vi "Main.vi"() -> ()   [LabVIEW 2013] (continued)
                                frame True {
                                # "Both FHS"
                                n2888 = Build Array(w4843, w4842) -> (w4844:refnum<vi>[])
                                }
                                }
                                n2889 = control-ref of="MCListBox FHS Setup Remove Button"() -> (w4836:refnum<vi>)
                                n2890 = control-ref of="MCListBox FHS Setup Add Button"() -> (w4837:refnum<vi>)
                                n2891 = local write "Edit WPS in Setup"(w4830) -> ()
                                n2892 = control-ref of="Tab Setup"() -> (w4839:refnum<vi>)
                                n2893 = local read "CellBG New Cells"() -> (w4832:u32)
                                n2894 = for {
                                tunnel: w4832 -> [w4849]
                                tunnel: w4835 -> [w4846] mode=indexing
                                # "MClistbox FHS Setup \nis set to FALSE for\n\"Allowing Editing Cells\"\n/\"Editable Cells"
                                # "Create WHITE\neditable cells"
                                n2895 = property on="Property Node" class="MCListbox (strict)"(reference=w4846, "Allow Editing Cells"=TRUE) -> (reference out=w4848:refnum<vi>, "NumCols"=w4847:u32)  [unwired: 1 in, 1 out]
                                n2896 = for {
                                N: w4847 -> [_]
                                tunnel: w4849 -> [w4851]
                                tunnel: w4848 -> [w4850]
                                i -> [w4853]
                                n2897 = Bundle("Multicolumn Listbox"=0, w4853) -> (w4852:cluster{"Multicolumn Listbox":i32, i32})  [unwired: 1 in]
                                n2898 = property on="Property Node" class="MCListbox (strict)"(reference=w4850, "ActiveCell"=w4852, "CellBG"=w4851) -> ()  [unwired: 1 in, 2 out]
                                }
                                }
                                n2899 = control-ref of="No."() -> (w4831:refnum<vi>)
                                n2900 = property class="Bool"(reference=w4836, "Visible"=w4830) -> ()  [unwired: 1 in, 2 out]
                                n2901 = property class="Bool"(reference=w4837, "Visible"=w4830) -> ()  [unwired: 1 in, 2 out]
                                n2902 = call "Setup Tab - Enable-Disable.vi"("No."=w4831, "[SRTRS][Config][ParameterSettings] - [userEditableProcedure]"=w4830, "Disabled"=T30."Enabled", "Tab Setup"=w4839) -> ()  [unwired: 8 in]
                              }
                            }
                            n2903 = call "DB - Convert BIT Type.vi"("BIT Type (eg Inactive)"=w4829) -> ("Boolean"=w4826:bool)  [unwired: 2 in, 2 out]
                          }
                          frame "ChartSeparation" {
                            # "Need DB - NA"
                            n2904 = call "DB - Convert BIT Type.vi"("BIT Type (eg Inactive)"=w4856) -> ("Boolean"=→"Chart Separation by Order#":bool)  [unwired: 2 in, 2 out]
                          }
                          frame "DataLogInterval" {
                            n2905 = Fract/Exp String To Number(string=w4858, default (0 dbl)=0.0) -> (number=w4860:dbl)  [unwired: 2 in, 1 out]
                            n2906 = local write "Host Sampling Interval (s)"(w4860) -> ()
                          }
                          frame "DateFormat" {
                            # "%<%H:%M:%S \n%Y-%m-%d>T"
                            n2907 = Empty String/Path?(string/path=w4862) -> (empty?=w4863:bool)
                            n2908 = case shown="False" w4863 {
                              tunnel: w4862 -> [w4868 _]
                              frame False {
                                # "We only fix time here. The date format is from DB"
                                # "Not Empty"
                                n2909 = Concatenate Strings("%<%H:%M:%S", "\n", w4868, ">T" ("string")) -> (w4867:string)
                                n2910 = property on="Chart" class="WFChart (strict)"("XScale.FormatString"=w4867) -> (error out=w4866:errorcluster)  [unwired: 2 in, 1 out]
                                n2911 = local write "Chart"(w4866) -> ()
                              }
                              frame True {
                                # "Empty"
                              }
                            }
                            "Date Format (UserDefined)" <- w4862
                          }
                          frame "EnableCmsUpdate" {
                            # "Need DB - NA"
                            n2912 = call "DB - Convert BIT Type.vi"("BIT Type (eg Inactive)"=w4873) -> ("Boolean"=w4872:bool)  [unwired: 2 in, 2 out]
                            "Enable Central Monitoring" <- w4872
                            n2913 = global write "Global SRTRS.vi" "Enable Central Monitoring"(w4872) -> ()
                          }
                          frame "EnableAmsUpdate" {
                            # "For Message UI"
                            # "No need to send to ini\nSince No DB, No AMS"
                            n2914 = call "DB - Convert BIT Type.vi"("BIT Type (eg Inactive)"=w4875) -> ("Boolean"=w4874:bool)  [unwired: 2 in, 2 out]
                            "Enable AMS Update" <- w4874
                            n2915 = global write "Global SRTRS.vi" "Enable AMS Update"(w4874) -> ()
                          }
                          frame "PermittedTempDiff" {
                            n2916 = Fract/Exp String To Number(string=w4877) -> (number=w4879:dbl)  [unwired: 3 in, 1 out]
                            n2917 = property on="Variant Allowed (Hold Temp)" class="DigNum (strict)"("Value"=w4879) -> ()  [unwired: 2 in, 2 out]
                          }
                          frame "PermittedTimeDiff" {
                            n2918 = Fract/Exp String To Number(string=w4881) -> (number=w4883:dbl)  [unwired: 3 in, 1 out]
                            n2919 = property on="Variant Allowed (Hold Time)" class="DigNum (strict)"("Value"=w4883) -> ()  [unwired: 2 in, 2 out]
                          }
                          frame "StartStopMarker" {
                            n2920 = call "DB - Convert BIT Type.vi"("BIT Type (eg Inactive)"=w4887) -> ("Boolean"=w4884:bool)  [unwired: 2 in, 2 out]
                            "Display Start Stop Marker" <- w4884
                          }
                          frame "DisplayRefChart" {
                            n2921 = call "DB - Convert BIT Type.vi"("BIT Type (eg Inactive)"=w4891) -> ("Boolean"=w4888:bool)  [unwired: 2 in, 2 out]
                            "Display Reference Chart" <- w4888
                          }
                        }
                        n2922 = case shown="\"String\"" w4798 {
                          tunnel: [w4815 w4823 w4825] -> w4804
                          tunnel: [w4814 w4822 w4824] -> w4797
                          tunnel: w4801 -> [w4813 w4821 w4825]
                          tunnel: w4803 -> [w4812 w4820 w4824]
                          tunnel: w4800 -> [w4811 w4818 _]
                          tunnel: w4799 -> [w4810 _ _]
                          tunnel: w4796 -> [_ w4817 _]
                          frame "String" {
                            n2923 = call-poly <vilib>:"Write Key.vi"("section"="Settings", "error in (no error)"=w4812, "value"=w4810, "key"=w4811, "refnum"=w4813) -> ("error out"=w4814:errorcluster, "refnum out"=w4815:T59)  [unwired: 4 in, 1 out]
                          }
                          frame "Boolean" {
                            n2924 = call-poly <vilib>:"Write Key.vi"("section"="Settings Boolean", "error in (no error)"=w4820, "value"=w4817, "key"=w4818, "refnum"=w4821) -> ("error out"=w4822:errorcluster, "refnum out"=w4823:T59)  [unwired: 4 in, 1 out]
                          }
                          frame "NA", Default {
                          }
                        }
                      }
                      n2925 = for {
                        tunnel: w4699 -> [w4760]
                        tunnel: w4698 -> [w4759]
                        tunnel: w4648 -> [w4757] mode=indexing
                        tunnel: [w4755] -> w4689
                        tunnel: [w4754] -> w4688
                        tunnel: w4709 -> [w4753]
                        tunnel: w4690 -> [w4752]
                        # "[Config].[GeneralSetting]"
                        n2926 = Format Into String(w4757) -> (resulting string=w4758:string)  [unwired: 3 in, 1 out]
                        n2927 = Search 1D Array(1D array=w4759, element=w4758) -> (index of element=w4761:i32)  [unwired: 1 in]
                        n2928 = Index Array(array=w4760, index=w4761) -> (element=w4756:string)
                        n2929 = case shown="\"TimeSyncSchedule\"" w4757 {
                          tunnel: w4756 -> [_ w4773 w4779 w4787 w4791]
                          tunnel: [_ "Log Off Timer" "cRIO Time Sync Schedule" "cRIO Time Sync Tolerance" _] -> w4751
                          tunnel: [_ w4773 w4779 w4787 _] -> w4750
                          tunnel: [_ Key_Enum."String" Key_Enum."String" Key_Enum."String" _] -> w4749
                          frame "GenericSystemId" {
                            # "Not in use"
                          }
                          frame "ScreenLockTimer" {
                            n2930 = Decimal String To Number(string=w4773) -> (number=w4776:i32)  [unwired: 2 in, 1 out]
                            n2931 = local write "Log Off Timer (s)"(w4776) -> ()
                          }
                          frame "TimeSyncSchedule" {
                            # "07:00"
                            n2932 = Match Pattern(string=w4779, regular expression=":") -> (before substring=w4783:string, after substring=w4782:string)  [unwired: 1 in, 2 out]
                            n2933 = Concatenate Strings(w4783, w4782) -> (w4781:string)
                            n2934 = Decimal String To Number(string=w4781) -> (number=w4778:i32)  [unwired: 2 in, 1 out]
                            n2935 = local write "cRIO Time Sync Schedule"(w4778) -> ()
                          }
                          frame "TimeSyncTolerance" {
                            # "60 (seconds)"
                            n2936 = Decimal String To Number(string=w4787) -> (number=w4786:i32)  [unwired: 2 in, 1 out]
                            n2937 = local write "cRIO Time Sync Tolerance"(w4786) -> ()
                          }
                          frame "TransactStartNo" {
                            # "No need to put in ini"
                            n2938 = Decimal String To Number(string=w4791) -> (number=w4790:i32)  [unwired: 2 in, 1 out]
                            "Starting Number for Transaction number" <- w4790
                            n2939 = Number To Decimal String(number=w4790) -> (decimal integer string=w4789:string)  [unwired: 1 in]
                            n2940 = global write "Global SRTRS.vi" "Transaction Start Number"(w4789) -> ()
                          }
                        }
                        n2941 = case shown="\"String\"" w4749 {
                          tunnel: [w4767 w4770 w4772] -> w4755
                          tunnel: [w4766 w4769 w4771] -> w4754
                          tunnel: w4753 -> [w4765 w4770 w4772]
                          tunnel: w4752 -> [w4764 w4769 w4771]
                          tunnel: w4751 -> [w4763 _ _]
                          tunnel: w4750 -> [w4762 _ _]
                          frame "String" {
                            n2942 = call-poly <vilib>:"Write Key.vi"("section"="Settings", "error in (no error)"=w4764, "value"=w4762, "key"=w4763, "refnum"=w4765) -> ("error out"=w4766:errorcluster, "refnum out"=w4767:T59)  [unwired: 4 in, 1 out]
                          }
                          frame "Boolean" {
                          }
                          frame "NA", Default {
                          }
                        }
                      }
                      n2943 = local read "SRTRS4070 Folder (Server Folder)"() -> (w4687:string)
                      n2944 = local read "SRTRS4070 Host Folder"() -> (w4686:string)
                      n2945 = local read "cRIO IP"() -> (w4685:string)
                      n2946 = global read "Global SRTRS.vi" "Temperature Units"() -> (w4684:string)
                      n2947 = local read "Plant and Furnace Name"() -> (w4683:string)
                      n2948 = local read "[LogoFile]"() -> (w4682:string)
                      n2949 = local read "ApplicationName"() -> (w4681:string)
                      n2950 = local read "Channel to Probe Mapping"() -> (w4680:cluster{"Channel to Probe Mapping":string})
                      n2951 = Unbundle By Name(w4680) -> ("Channel to Probe Mapping"=w4679:string)
                      n2952 = Build Array(w4687, w4686, w4685, w4684, w4683, w4682, w4681, w4679) -> (w4678:string[])
                      n2953 = control-ref of="Equipment Details"() -> (w4673:refnum<vi>)
                      n2954 = control-ref of="Furnace Details"() -> (w4675:refnum<vi>)
                      n2955 = for {
                        tunnel: w4689 -> [w4736]
                        tunnel: w4688 -> [w4735]
                        tunnel: [w4734] -> w4677
                        tunnel: [w4733] -> w4676
                        tunnel: w4678 -> [w4732] mode=indexing
                        tunnel: string[] ["SRTRS4070 Folder", "SRTRS4070 Host Folder", "cRIO IP", "Temperature Units", "Plant and Furnace Name", "LogoFile", "Software Solution Name", "Channel to Probe Mapping", ""] -> [w4731] mode=indexing
                        n2956 = case shown="\"String\"" Key_Enum."String" {
                          tunnel: [w4743 w4746 w4748] -> w4734
                          tunnel: [w4742 w4745 w4747] -> w4733
                          tunnel: w4736 -> [w4741 w4746 w4748]
                          tunnel: w4735 -> [w4740 w4745 w4747]
                          tunnel: w4731 -> [w4739 _ _]
                          tunnel: w4732 -> [w4738 _ _]
                          frame "String" {
                            n2957 = call-poly <vilib>:"Write Key.vi"("write raw string? (F)"=TRUE, "section"="Settings", "error in (no error)"=w4740, "value"=w4738, "key"=w4739, "refnum"=w4741) -> ("error out"=w4742:errorcluster, "refnum out"=w4743:T59)  [unwired: 3 in, 1 out]
                          }
                          frame "Boolean" {
                          }
                          frame "NA", Default {
                          }
                        }
                      }
                      n2958 = call "Key - Cluster Write.vi"("error in (no error)"=w4676, "Cluster Ref in"=w4675, "Refnum in"=w4677) -> ("error out"=w4671:errorcluster, "Refnum out"=w4672:T59)  [unwired: 7 in]
                      n2959 = call "Key - MCListbox Write.vi"("Remove \\r\\n"=TRUE ("Remove \\r\\n"), "delimiter (,)"="\t", "error in (no error)"=w4671, "MulticolumnListbox Ref in"=w4673, "refnum"=w4672) -> ("error out"=w4658:errorcluster, "Refnum out"=w4659:T59)  [unwired: 3 in, 2 out]
                      n2960 = call <vilib>:"Close Config Data.vi"("error in (no error)"=w4658, "refnum"=w4659) -> ("error out"=w4660:errorcluster)  [unwired: 8 in, 1 out]
                      n2961 = local write "ini File Error"(w4660) -> ()
                    }
                    frame 2.. {
                      (unwired) string[] ["OrderNo", "OperationNo", "Qty", "NCRNo", "CustomerID", "Customer", "Project", "SalesOrderNo", "SalesOrderItemNo", "MaterialNo", "MaterialRev", "MaterialDesc", "SerialNos", "UnitOfQty"]  # 2014-10-17 08:39 [Config].[Mapping].[ColumnName]
                      w4898 = string[] ["Order No.", "Oper. No.", "Qty.", "NCR No.", "Customer No.", "Customer Name", "Project", "Sales Order", "Item No.", "Material", "Revision", "Material Description", "Serial No.", "UnitOfQty"]  # 2014-10-17 08:39 Item Details Label.Text
                      # "SubVI VI's Path\n..\\SRTRS\\VIs\\SubVIs\\DB UI - Calibration History.vi\nOR \n..\\SRTRS\\SRTRS.exe\\SubVIs\\DB UI - Calibration History.vi"
                      # "[Config].[Mapping].[ColumnName]"
                      # "SubPanel VI's Path\n..\\SRTRS\\VIs\\SubPanels\\DB UI - Logon.vi\nOR \n..\\SRTRS\\SRTRS.exe\\SubPanels\\DB UI - Logon.vi"
                      # "Current VI's Path\n..\\SRTRS\\VIs\\Main.vi\nOR \n..\\SRTRS\\SRTRS.exe\\Main.vi"
                      n2962 = local read "Logon"() -> (w4904:T21)
                      n2963 = local read "Update English Captions"() -> (w4892:bool)
                      n2964 = Unbundle By Name(w4904) -> ("LanguageID"=w4903:string)
                      n2965 = To Upper Case(1:w4903) -> (0:w4901:string)
                      n2966 = Not Equal?(x=w4901, y="EN") -> (x != y?=w4894:bool)
                      n2967 = Or(x=w4892, y=w4894) -> (x .or. y?=w4893:bool)
                      n2968 = case shown="True" w4893 {
                        tunnel: w4901 -> [_ w4924]
                        tunnel: [_ errorcluster {"status"=FALSE, "code"=0, "source"=""} ("error constant")] -> w4895
                        frame False {
                        }
                        frame True {
                          n2969 = case shown="True" "Dummy Load" {
                            tunnel: [_ w4927] -> w4922
                            frame False {
                            }
                            frame True {
                              # "\"Load with Callers\"but will not be Run here.\nWe need to Load otherwise cannot set Caption from Main.vi \nBecause this is called by SubPanel, i.e. 2 levels down."
                              n2970 = call "DB UI - Calibration History.vi"() -> ("SUMMARY"=w4927:errorcluster)  [unwired: 10 in, 1 out]
                            }
                          }
                          n2971 = for {
                            tunnel: [w4933] -> w4925
                            tunnel: w4924 -> [w4929]
                            tunnel: string[] ["Main.vi", "SubVIs\\DB UI - Calibration History.vi", "SubVIs\\DB UI - MasterData SAPMaterial (Long) Description.vi", "SubVIs\\DB UI - MasterData SAPProduction Long Text.vi", "SubVIs\\DB UI - Search-Load Setup.vi", "SubVIs\\DB UI - Transaction Details.vi"] -> [w4928] mode=indexing
                            tunnel: w4922 -> [_]
                            n2972 = local read "Current VI's path"() -> (w4935:path)
                            n2973 = control-ref of="MasterData\\Language"() -> (w4932:refnum<vi>)
                            n2974 = call "String - Create Caption Paths.vi"("LanguageID"=w4929, "name or relative path"=w4928, "Current VI's path"=w4935, "Path in"=w4932) -> ("xml Path"=w4930:path, "VI Path"=w4934:path)  [unwired: 6 in]
                            n2975 = call "Caption Main VI.vi"("Read/Write(T) XML"=FALSE, "Read xml path"=w4930, "VI path"=w4934) -> ("Error Out"=w4933:errorcluster)  [unwired: 8 in]
                          }
                          "Caption Error Out" <- w4925
                        }
                      }
                      n2976 = control-ref of="Item Details"() -> (w4900:refnum<vi>)
                      n2977 = local read "[IsMandatory]"() -> (w4896:string[])
                      n2978 = flat-sequence "Also Called in Tab Value Change (Report)" {
                        frame #0 {
                          w4916 = 60 ("y")
                          # "Initialize Report Tab"
                          n2979 = disable-structure shown="Disabled" {
                            frame Disabled {
                              w4920 = ""
                              n2980 = property on="Selection Transaction No" class="CmbBox (strict)"("Value"=w4920) -> ()  [unwired: 2 in, 2 out]
                              n2981 = property on="Selection Order No" class="CmbBox (strict)"("Value"=w4920) -> ()  [unwired: 2 in, 2 out]
                            }
                            frame Enabled {
                            }
                          }
                          n2982 = Get Date/Time In Seconds() -> (seconds since 1Jan1904=w4919:timestamp)
                          n2983 = Multiply(x=7, y=24) -> (x*y=w4914:i32)
                          n2984 = Format Date/Time String(time format string (%c)="%m") -> (date/time string=w4907:string)  [unwired: 2 in]
                          n2985 = Format Date/Time String(time format string (%c)="%Y") -> (date/time string=w4908:string)  [unwired: 2 in]
                          n2986 = Multiply(x=w4914, y=w4916) -> (x*y=w4915:i32)
                          n2987 = Multiply(x=w4915, y=w4916) -> (x*y=w4917:i32)
                          n2988 = Decimal String To Number(string=w4908) -> (number=w4909:i32)  [unwired: 2 in, 1 out]
                          n2989 = Decimal String To Number(string=w4907) -> (number=w4906:i32)  [unwired: 2 in, 1 out]
                          n2990 = Subtract(x=w4919, y=w4917) -> (x-y=w4918:timestamp)
                          n2991 = property on="Date End" class="AbsTime (strict)"("Value"=w4919) -> ()  [unwired: 2 in, 2 out]
                          n2992 = property on="Date Start" class="AbsTime (strict)"("Value"=w4918) -> ()  [unwired: 2 in, 2 out]
                          n2993 = local write "FTP Year"(w4909) -> ()
                          n2994 = local write "FTP Month"(w4906) -> ()
                          n2995 = property on="Report Open" class="Bool"("DisabledEnum"=T30."Disabled and Grayed Out" ("Disabled")) -> ()  [unwired: 2 in, 2 out]
                        }
                      }
                      n2996 = property class="Clust (strict)"(reference=w4900, error in=w4895) -> ("Controls[]"=w4899:refnum<vi>[])  [unwired: 2 out]
                      n2997 = for {
                        tunnel: w4899 -> [w4943] mode=indexing
                        tunnel: w4898 -> [w4942]
                        tunnel: w4896 -> [w4941]
                        tunnel: [w4937] -> w4897 mode=indexing if=w4936
                        # "Look for Mandatory Fields and put * at end of Caption"
                        n2998 = property class="Ctl"(reference=w4943) -> (reference out=w4939:refnum<vi>, "Label.Text"=w4938:string)  [unwired: 1 in, 1 out]
                        n2999 = Search 1D Array(1D array=w4942, element=w4938) -> (index of element=w4940:i32)  [unwired: 1 in]
                        n3000 = case shown="0, Default" w4940 {
                          selector: w4940 -> [w4960 _]
                          tunnel: w4941 -> [w4962 _]
                          tunnel: w4939 -> [w4959 _]
                          tunnel: w4938 -> [w4950 _]
                          tunnel: [w4949 ""] -> w4937
                          tunnel: [w4948 FALSE] -> w4936
                          frame 0, Default {
                            # "Remove all * or * (unicode) in caption"
                            # "Found Control"
                            n3001 = Index Array(array=w4962, index=w4960) -> (element=w4961:string)
                            n3002 = call "DB - Convert BIT Type.vi"("BIT Type (eg Inactive)"=w4961) -> ("Boolean"=w4948:bool)  [unwired: 2 in, 2 out]
                            n3003 = property class="Ctl"(reference=w4959) -> (reference out=w4955:refnum<vi>, "Caption.Text"=w4956:string, "Caption.Left"=w4954:i32)  [unwired: 1 in, 1 out]
                            n3004 = Search and Replace String(replace all?=TRUE ("replace all? (F)"), input string=w4956, search string="*\u0000") -> (result string=w4947:string)  [unwired: 5 in, 3 out]
                            n3005 = Search and Replace String(replace all?=TRUE ("replace all? (F)"), input string=w4947, search string="*") -> (result string=w4946:string)  [unwired: 5 in, 3 out]
                            n3006 = case shown="True" w4948 {
                              tunnel: w4946 -> [w4965 w4968]
                              tunnel: w4955 -> [w4966 w4978]
                              tunnel: w4954 -> [w4964 w4976]
                              tunnel: [w4966 w4978] -> w4953
                              tunnel: [w4965 w4977] -> w4952
                              tunnel: [w4964 w4976] -> w4951
                              tunnel: w4950 -> [_ w4975]
                              tunnel: ["" w4975] -> w4949
                              frame False {
                                # "Removes * in Caption"
                              }
                              frame True {
                                # "Check if Multibyte"
                                # "IsMandatory, add *"
                                n3007 = String Subset(string=w4968, length (rest)=2 ("length (rest)")) -> (substring=w4970:string)  [unwired: 1 in]
                                n3008 = Equal?(x=w4970, y="ÿþ") -> (x = y?=w4967:bool)
                                n3009 = Select(t="*\u0000" ("string"), s=w4967, f="*" ("string")) -> (s? t:f=w4973:string)
                                n3010 = Concatenate Strings(w4968, w4973) -> (w4977:string)
                              }
                            }
                            n3011 = property class="Ctl"(reference=w4953, "Caption.Text"=w4952, "Caption.Left"=w4951) -> ()  [unwired: 1 in, 2 out]
                          }
                          frame -1 {
                          }
                        }
                      }
                      "[IsMandatory]\nLabel.Text" <- w4897
                    }
                  }
                }
              }
            }
          }
          frame "Execute", Default {
            # "DAQ Started OR RecoveryFlag?"
            # "All Pages Except LOGON"
            n3012 = case shown="\"Setup\", Default" w4981 {
              tunnel: [FALSE ("Time has Elapsed") w4989] -> w4982
              frame "Setup", Default {
                # "Resets cRIO Check Time Target\nif we are not in the EXECUTE\nTab"
                n3013 = local write "Time Target (s)"(0.0 ("Time Target (s)")) -> ()
              }
              frame "Execute" {
                # "Only Check if Execute Tab"
                n3014 = call "Elapsed Time"("Time Target (s)"="Time Target (s)") -> ("Time has Elapsed"=w4989:bool)  [unwired: 11 in, 7 out]
              }
            }
            n3015 = First Call?() -> (First Call?: T/F=w4983:bool)
            n3016 = case shown="True" w4982 {
              tunnel: [w5011 w5127] -> w4986
              tunnel: [w5012 w5096] -> w4985
              tunnel: [errorcluster {"status"=FALSE, "code"=0, "source"=""} ("error IO") w5110] -> w4984
              frame False {
                (unwired) 70000 ("upper limit")
                w5011 = 0  # Sample/ch Count
                w5012 = FALSE  # Not Checking DAQ Started/Recovery here
                # "1st time this should be blank"
                # "Only Date is Used\nCheck Once per day"
                # "1 min window"
                # "Not Checking Status of cRIO and ET,\nSo we check TimeSync"
                n3017 = local read "Day cRIO Time is SET"() -> (w4995:string)
                n3018 = global read "Global SRTRS.vi" "Logon"() -> (w5001:T21)
                n3019 = global read "Global SRTRS.vi" "Date Format"() -> (w5006:string)
                n3020 = local read "cRIO Time Sync Schedule"() -> (w4992:i32)
                n3021 = local read "Day cRIO Time is SET"() -> (w5004:string)
                n3022 = Unbundle By Name(w5001) -> ("StationID"=w5000:string)
                n3023 = disable-structure shown="Disabled" {
                  frame Disabled {
                    n3024 = local read "Logon OK"() -> ()  [unwired: 1 out]
                  }
                  frame Enabled {
                  }
                }
                n3025 = Format Date/Time String(time format string (%c)="%H%M%S") -> (date/time string=w5008:string)  [unwired: 2 in]
                n3026 = Format Date/Time String(time format string (%c)=w5006) -> (date/time string=w5005:string)  [unwired: 2 in]
                n3027 = Decimal String To Number(string=w5008) -> (number=w5007:i32)  [unwired: 2 in, 1 out]
                n3028 = String Length(string=w5000) -> (length=w4999:i32)
                n3029 = Empty String/Path?(string/path=w4995) -> (empty?=w4994:bool)
                n3030 = Add(x=100 ("upper limit"), y=w4992) -> (x+y=w4991:i32)
                n3031 = Not Equal?(x=w5005, y=w5004) -> (x != y?=w5002:bool)
                n3032 = Greater Than 0?(x=w4999) -> (x > 0?=w4998:bool)
                n3033 = In Range and Coerce(upper limit=w4991, x=w5007, lower limit=w4992) -> (In Range?=w4997:bool)  [unwired: 1 out]
                n3034 = Or(x=w4997, y=w4994) -> (x .or. y?=w4996:bool)
                n3035 = Compound Arithmetic op=AND(w4996, w5002, w4998) -> (w5003:bool)
                n3036 = case shown="True" w5003 {
                  tunnel: [_ w5041] -> _
                  tunnel: w5005 -> [_ w5034]
                  frame False {
                  }
                  frame True {
                    (unwired) Message_Code_-_Enum."<APP><I 100>" ("Message Code\n2014-10-01")
                    # "070000 to 070100"
                    n3037 = local read "cRIO shared variable RT Library"() -> (w5036:string)
                    n3038 = local read "Simulate cRIO"() -> (w5035:bool)
                    n3039 = control-ref of="cRIO Status"() -> (w5038:refnum<vi>)
                    n3040 = call "cRIO - Shared Variable RW.vi"("shared variable RT Library"=w5036, "Read/Write"=cRIO_RW_Enum."Read", "Simulate cRIO"=w5035, "cRIO Status"=w5038) -> ("cRIO Timestamp"=w5032:timestamp, "DAQ Started"=w5024:bool, "Error Out"=w5039:errorcluster)  [unwired: 7 in, 6 out]
                    n3041 = local read "cRIO Time Sync Tolerance"() -> (w5014:i32)
                    n3042 = local write "cRIO DAQ Started"(w5024) -> ()
                    n3043 = Get Date/Time In Seconds() -> (seconds since 1Jan1904=w5033:timestamp)
                    n3044 = Unbundle By Name(w5039) -> ("status"=w5040:bool)
                    n3045 = Select(t="cRIO DAQ Started. " ("format string"), s=w5024, f="cRIO DAQ NOT Started. " ("format string")) -> (s? t:f=w5017:string)
                    n3046 = Subtract(x=w5033, y=w5032) -> (x-y=w5031:dbl)
                    n3047 = Not(x=w5040) -> (.not. x?=w5019:bool)
                    n3048 = Select(t="cRIO Comm GOOD. " ("format string"), s=w5019, f="cRIO Comm Error. " ("format string")) -> (s? t:f=w5018:string)
                    n3049 = Absolute Value(x=w5031) -> (abs(x)=w5025:dbl)
                    n3050 = Format Into String(format string="{Ready to Start} Time Difference is %d seconds. ", w5025) -> (resulting string=w5016:string)  [unwired: 2 in, 1 out]
                    n3051 = Concatenate Strings(w5016, w5017, w5018) -> (w5013:string)
                    n3052 = Not(x=w5024) -> (.not. x?=w5030:bool)
                    n3053 = Greater?(x=w5025, y=w5014) -> (0:w5027:bool)
                    n3054 = call "Queue - EnQueue to MessageQ.vi"("<NoD> Don't Display to UI"=TRUE, "Message"=w5013) -> ("Error Out"=w5015:errorcluster)  [unwired: 9 in]
                    n3055 = Compound Arithmetic op=AND(w5027, w5030, w5019) -> (w5029:bool)
                    n3056 = case shown="True" w5029 {
                      tunnel: [_ w5044] -> w5041
                      tunnel: w5035 -> [_ w5043]
                      tunnel: w5033 -> [_ w5042]
                      tunnel: w5015 -> [_ _]
                      frame False {
                      }
                      frame True {
                        # "cRIO DAQ NOT Started AND NO ERROR"
                        n3057 = case shown="True" w5043 {
                          tunnel: [w5049 _] -> w5044
                          tunnel: w5042 -> [w5054 _]
                          frame False {
                            w5056 = u32 300000  # remote timeout in ms (5min)
                            # "If we are using \"time zone\" string:\nTime Zone strings need to be of the form Etc/GMT-X or Etc/GMT+X where X represents the offset from GMT. For example Etc\\GMT-6 is the equivalent to Central Standard Time in the US. (GMT-5 during Daylight Saving Time). Valid values range from 12 to -13 centered around GMT."
                            # "Time Difference > 60s AND\ncRIO DAQ NOT Started AND\ncRIO Comm no Error"
                            n3058 = flat-sequence {
                              tunnel: [errorcluster {"status"=FALSE, "code"=0, "source"=""} ("error in (no error)")] -> w5053
                              frame #0 {
                                # "120 seconds wait"
                                n3059 = call "Msgbox - Add OR Remove.vi"("MsgBox"=T44 {"Show"=TRUE, "Priority"=0, "Message"="Setting cRIO Clock...", "seconds"=120}) -> ()  [unwired: 9 in, 2 out]
                              }
                            }
                            n3060 = local read "cRIO IP"() -> (w5058:string)
                            n3061 = case shown="True" FALSE {
                              tunnel: w5054 -> [w5084 w5086]
                              tunnel: [w5084 w5085] -> w5057
                              frame False {
                              }
                              frame True {
                                # "UTC-7 hours"
                                n3062 = Multiply(x=60, y=60) -> (x*y=w5089:i32)
                                n3063 = Multiply(x=w5089, y=7) -> (x*y=w5087:i32)
                                n3064 = Subtract(x=w5086, y=w5087) -> (x-y=w5085:timestamp)
                              }
                            }
                            n3065 = call <vilib>:"Initialize Session.vi"("connect timeout in ms (4s)"=u32 5000, "error in (no error)"=w5053, "force property refresh (T)"=TRUE, "target (localhost)"=w5058) -> ("error out"=w5062:errorcluster, "session out"=w5063:refnum<k21>)  [unwired: 6 in]
                            n3066 = call <vilib>:"Set Time.vi"("remote timeout in ms (5m)"=w5056, "error in (no error)"=w5062, "time"=w5057, "session in (localhost)"=w5063) -> ("error out"=w5061:errorcluster, "session out"=w5064:refnum<k21>)  [unwired: 4 in, 2 out]
                            n3067 = call-poly <vilib>:"Close.vi"("error in (no error)"=w5061, "session in"=w5064) -> ("error out"=w5051:errorcluster)  [unwired: 9 in]
                            n3068 = flat-sequence {
                              tunnel: w5051 -> [w5081]
                              tunnel: [w5079] -> w5048
                              tunnel: [w5073] -> w5050
                              tunnel: w5050 -> [w5082]
                              tunnel: [w5082] -> w5049
                              frame #0 {
                                # "Check SYNC"
                                # "For Folder Management\non cRIO"
                                n3069 = local read "cRIO Time Sync Tolerance"() -> (w5069:i32)
                                n3070 = local read "cRIO shared variable RT Library"() -> (w5072:string)
                                n3071 = Concatenate Strings(w5072, "/cRIO Timestamp" ("string")) -> (w5070:string)
                                n3072 = call "cRIO - Check Time Sync.vi"("Error In"=w5081, "Time Sync Tolerance (60sec)"=w5069, "Timeout (minutes)"=2, "cRIO Timestamp SV"=w5070) -> ("error out 4"=w5074:errorcluster, "cRIO Timestamp SYNCed"=w5079:bool)  [unwired: 4 in, 2 out]
                                n3073 = control-ref of="cRIO Status"() -> (w5076:refnum<vi>)
                                n3074 = local read "cRIO Data Retention"() -> (w5078:i32)
                                n3075 = local read "Simulate cRIO"() -> (w5075:bool)
                                n3076 = call "cRIO - Shared Variable RW.vi"("shared variable RT Library"=w5072, "Read/Write"=cRIO_RW_Enum."Write Others", "Error In"=w5074, "Simulate cRIO"=w5075, "cRIO Data Retention"=w5078, "cRIO Status"=w5076) -> ("Error Out"=w5073:errorcluster)  [unwired: 5 in, 8 out]
                              }
                              frame #1 {
                                n3077 = call "Msgbox - Add OR Remove.vi"("MsgBox"=T44 {"Show"=FALSE, "Priority"=0, "Message"="Setting cRIO Clock...(Done)", "seconds"=120}) -> ()  [unwired: 9 in, 2 out]
                              }
                            }
                            n3078 = case shown="True" w5048 {
                              tunnel: ["cRIO Set Time Failed." ("Message") "cRIO TIme Sync OK." ("Message")] -> w5047
                              frame False {
                              }
                              frame True {
                              }
                            }
                            n3079 = Concatenate Strings("{Ready to Start}" ("Message"), w5047) -> (w5045:string)
                            n3080 = call "Queue - EnQueue to MessageQ.vi"("<NoD> Don't Display to UI"=TRUE, "Message"=w5045) -> ()  [unwired: 9 in, 1 out]
                          }
                          frame True {
                            # "Simulate cRIO"
                            n3081 = call "Queue - EnQueue to MessageQ.vi"("<NoD> Don't Display to UI"=TRUE, "Message"="{Ready To Start} Simulate cRIO Set Time.") -> ()  [unwired: 9 in, 1 out]
                          }
                        }
                      }
                    }
                    "Day cRIO Time is SET" <- w5034
                  }
                }
              }
              frame True {
                w5094 = TRUE  # Skip TimeStamps
                # "Does NOT Work in Simulation unless cRIO DAQ Started is TRUE"
                # "No need to update DB here. \n[SRTRS].[Execute].[TransactionResult] record not created yet \n[CMS].[Execute].[ActiveProcess] IsActve is F, so don't update"
                # "cRIO Already Started, SET Recovery Flag"
                # "Check cRIO and ET Status"
                n3082 = local write "Time Target (s)"(10.0 ("Time Target (s)")) -> ()
                n3083 = local read "cRIO shared variable RT Library"() -> (w5129:string)
                n3084 = local read "VISA resource name RS232"() -> (w5125:string)
                n3085 = control-ref of="cRIO Status"() -> (w5107:refnum<vi>)
                n3086 = control-ref of="ET3504 Status"() -> (w5098:refnum<vi>)
                n3087 = call "cRIO - Shared Variable RW.vi"("shared variable RT Library"=w5129, "Read/Write"=cRIO_RW_Enum."Read", "Simulate cRIO"="Simulate cRIO", "cRIO Status"=w5107) -> ("Probe List Out"=w5120:i32[], "cRIO Timestamp"=→"cRIO Timestamp":timestamp, "Data Path Name"=w5108:string, "Cycle Count"=w5127:i32, "DAQ Started"=w5096:bool, "Error Out"=w5102:errorcluster)  [unwired: 7 in, 3 out]
                "cRIO DAQ Started" <- w5096
                "cRIO Cycle Count" <- w5127
                "cRIO Error" <- w5102
                n3088 = call "ET3500 - Read Program Parameters.vi"("Simulate"="Simulate ET3500", "ET3500 Status"=w5098, "error in (no error)"=w5102, "subVI (Auto Interactive)"=TRUE ("subVI"), "Option"=cluster{"Init":bool, "Close":bool} {"Init"=TRUE, "Close"=TRUE}, "VISA resource name"=w5125) -> ("error out"=w5115:errorcluster, "Segment.Type"=w5114:i16, "Parameter Cluster (Scaled)"=w5113:T76)  [unwired: 1 in, 2 out]
                "ET3500 Error" <- w5115
                n3089 = Unbundle By Name(w5113) -> ("PVIn (degC)"=w5119:dbl)
                n3090 = local write "Data Path Name (cRIO SV)"(w5108) -> ()
                n3091 = case shown="True" w5096 {
                  tunnel: [FALSE w5132] -> w5109
                  frame False {
                  }
                  frame True {
                    n3092 = local read "DB - Transaction"() -> (w5131:bool)
                    n3093 = case shown="True" w5131 {
                      tunnel: [w5133 w5150] -> w5132
                      frame False {
                        # "Use ini file\nRaw Data File should have the uncompleted Raw Data FIle from last [TransactionNo] and [TransactionRunNo]"
                        n3094 = local read "Raw Data File"() -> (w5135:string)
                        n3095 = Empty String/Path?(string/path=w5135) -> (empty?=w5134:bool)
                        n3096 = Not(x=w5134) -> (.not. x?=w5133:bool)
                      }
                      frame True {
                        # "Use DB\nCheck Existing [TransactionNo]/[TransactionRunNo]  in [Execute].[Active]"
                        n3097 = global read "Global SRTRS.vi" "Logon"() -> (w5147:T21)
                        n3098 = Unbundle By Name(w5147) -> ("PlantID"=w5146:string, "StationID"=w5145:string)
                        n3099 = Build Array(w5146, w5145) -> (w5144:string[])
                        n3100 = call "DB - [Execute].[Transaction].vi"("DB.Schema.Table"="SRTRS.Execute.Active", "DB - Execute Transaction"=DB_-_Execute_Transaction_Enum."SELECT [Execute].[Active]", "<Values>"=w5144) -> ("1D Results"=w5143:string[], "SUMMARY"=w5136:errorcluster)  [unwired: 13 in, 2 out]
                        n3101 = local write "DB"(w5136) -> ()
                        n3102 = Index Array(array=w5143) -> (element #1=w5140:string, element #2=w5142:string)  [unwired: 2 in]
                        n3103 = local write "TransactionRunNo (Execute)"(w5142) -> ()
                        n3104 = global write "Global SRTRS.vi" "[TransactionRunNo]"(w5142) -> ()
                        n3105 = local write "Transaction No (Execute)"(w5140) -> ()
                        n3106 = global write "Global SRTRS.vi" "[TransactionNo]"(w5140) -> ()
                        n3107 = local write "TransactionRunNo"(w5142) -> ()
                        n3108 = local write "Transaction No"(w5140) -> ()
                        n3109 = Empty String/Path?(string/path=w5140) -> (empty?=w5139:bool)
                        n3110 = Empty String/Path?(string/path=w5142) -> (empty?=w5141:bool)
                        n3111 = Not "IsNotEmpty"(x=w5139) -> (.not. x?=w5138:bool)
                        n3112 = Not "IsNotEmpty"(x=w5141) -> (.not. x?=w5137:bool)
                        n3113 = And(x=w5138, y=w5137) -> (x .and. y?=w5150:bool)
                        n3114 = property on="TransactionRunNo" class="Str"("Visible"=w5150) -> ()  [unwired: 2 in, 2 out]
                      }
                    }
                  }
                }
                n3115 = global read "Global SRTRS.vi" "Logon"() -> (w5106:T21)
                n3116 = control-ref of="MCListBox FHS Setup"() -> (w5117:refnum<vi>)
                n3117 = Unbundle By Name(w5106) -> ("PlantID"=w5104:string, "SystemID"=w5105:string)
                n3118 = control-ref of="WPS Details Setup"() -> (w5111:refnum<vi>)
                n3119 = property on="Current Temp" class="DigNum (strict)"("Value"=w5119) -> ()  [unwired: 2 in, 2 out]
                n3120 = control-ref of="Sequence Status"() -> (w5116:refnum<vi>)
                n3121 = Bundle("PlantID"=w5104, "SystemID"=w5105) -> (w5103:cluster{"PlantID":string, "SystemID":string})  [unwired: 1 in]
                n3122 = Merge Errors(w5115, w5102) -> (w5110:errorcluster)
                n3123 = case shown="True" w5096 {
                  tunnel: w5120 -> [_ w5193]
                  frame False {
                    # "Probe List not loaded yet"
                  }
                  frame True {
                    # "DAQ Started, Probe already Loaded in"
                    n3124 = local write "Probe List"(w5193) -> ()
                  }
                }
                n3125 = call "Status - Update cRIO Status.vi"("Skip TimeStamps"=w5094, "Error In"=w5102, "[PlantId],[SystemId]"=w5103, "cRIO Status"=w5107) -> ("Error Out"=w5100:errorcluster)  [unwired: 7 in]
                n3126 = call "Status - Update Sequence Status.vi"("Sequence Status"=w5116, "WPS Details"=w5111, "DB - Transaction"=FALSE, "MCListBox FHS Setup"=w5117, "ET3504 Status"=w5098, "Error In"=w5115, "Parameter Cluster (Scaled)"=w5113, "DB - Active Process"=FALSE, "Segment.Type"=w5114) -> ("Error Out"=w5101:errorcluster)  [unwired: 5 in, 1 out]
                n3127 = local write "Parameter Cluster (Scaled)"(w5113) -> ()
                n3128 = Merge Errors(w5101, w5100) -> (w5099:errorcluster)
                n3129 = local write "System Status"(w5099) -> ()
                n3130 = And(x=w5096, y=w5109) -> (x .and. y?=w5095:bool)
                n3131 = case shown="True" w5095 {
                  frame False {
                  }
                  frame True {
                    # "Either cRIO already Started OR\nExisting [TransactionNo]/[TransactionRunNo] in [Execute].[Active]"
                    # "Recovery"
                    n3132 = local read "DB - Setup Item (Part Details)"() -> (w5159:bool)
                    n3133 = case shown="False" w5159 {
                      frame False {
                        # "Lastest stp file was loaded at the beginning\nof the program."
                        # "Recovered from SRTRS.ini file"
                        # "Use File"
                        n3134 = local read "Latest stp file"() -> (w5162:path)
                        n3135 = call <vilib>:"Check if File or Folder Exists.vi"("path"=w5162) -> ("file or folder exists?"=w5161:bool, "dup path"=w5160:path)  [unwired: 8 in, 1 out]
                        n3136 = case shown="True" w5161 {
                          tunnel: w5160 -> [_ w5187]
                          frame False {
                          }
                          frame True {
                            n3137 = Strip Path(path=w5187) -> (name=w5188:string)  [unwired: 1 out]
                            n3138 = control-ref of="WPS Details Buffer"() -> (w5173:refnum<vi>)
                            n3139 = Match Pattern(string=w5188, regular expression="_") -> (before substring=w5163:string)  [unwired: 1 in, 3 out]
                            n3140 = call <vilib>:"Open Config Data.vi"("create file if necessary (T)"=FALSE, "configuration file path"=w5187) -> ("error out"=w5183:errorcluster, "refnum"=w5185:T59)  [unwired: 7 in, 1 out]
                            n3141 = control-ref of="WPS Details Setup"() -> (w5184:refnum<vi>)
                            n3142 = local write "Transaction No (Execute)"(w5163) -> ()
                            n3143 = global write "Global SRTRS.vi" "[TransactionNo]"(w5163) -> ()
                            n3144 = local write "Transaction No"(w5163) -> ()
                            n3145 = call "Key - Cluster Read.vi"("error in (no error)"=w5183, "New Ctl Ref"=w5173, "Original Ctl Ref"=w5184, "Refnum in"=w5185) -> ("error out"=w5170:errorcluster, "Refnum out"=w5171:T59)  [unwired: 5 in, 1 out]
                            n3146 = control-ref of="Parameter Buffer"() -> (w5169:refnum<vi>)
                            n3147 = call "Key - Cluster Read.vi"("error in (no error)"=w5170, "New Ctl Ref"=w5169, "Original Ctl Ref"=w5169, "Refnum in"=w5171) -> ("error out"=w5166:errorcluster, "Refnum out"=w5168:T59)  [unwired: 5 in, 1 out]
                            n3148 = control-ref of="Final Target Temperature"() -> (w5164:refnum<vi>)
                            n3149 = call "Key - Cluster Read.vi"("error in (no error)"=w5166, "New Ctl Ref"=w5164, "Original Ctl Ref"=w5164, "Refnum in"=w5168) -> ("error out"=w5165:errorcluster, "Refnum out"=w5167:T59)  [unwired: 5 in, 1 out]
                            n3150 = call <vilib>:"Close Config Data.vi"("error in (no error)"=w5165, "write file if changed (T)"=FALSE, "refnum"=w5167) -> ("error out"=w5172:errorcluster)  [unwired: 7 in, 1 out]
                            n3151 = local write "stp file Error Out"(w5172) -> ()
                            n3152 = property class="Clust (strict)"(reference=w5173, error in=w5172) -> (error out=w5174:errorcluster, "Value"=w5181:T28)  [unwired: 1 out]
                            n3153 = Unbundle By Name(w5181) -> ("WPS/Ref"=w5177:T5, "WPS Details Temperature Units"=w5178:string, "Hold Temperature"=w5179:string, "Hold Time (HH:MM)"=w5180:string)
                            n3154 = local write "Property Node Error"(w5174) -> ()
                            n3155 = local read "Info."() -> (w5175:T9)
                            n3156 = Bundle By Name(cluster=w5175, "Ref WPS"=w5177, "Info. Temperature Units"=w5178, "Info. Temperature Units 2"=w5178, "Hold. Temp."=w5179, "Hold. Time (hour:minute)"=w5180) -> (w5176:T9)
                            n3157 = local write "Info."(w5176) -> ()
                          }
                        }
                      }
                      frame True {
                        # "Use DB"
                        n3158 = flat-sequence {
                          frame #0 {
                            # "We are doing a auto reload of Setup Parameters"
                            n3159 = property on="Search Setup Toggle" class="Bool (strict)"() -> ("Value"=w5192:bool)  [unwired: 2 in, 2 out]
                            n3160 = Not(x=w5192) -> (.not. x?=w5191:bool)
                            n3161 = property on="Search Setup Toggle" class="Bool (strict)"("Val(Sgnl)"=w5191) -> ()  [unwired: 2 in, 2 out]
                          }
                        }
                        n3162 = property on="Recipe Stop" class="Bool"("DisabledEnum"=T30."Enabled" ("Disabled")) -> ()  [unwired: 2 in, 2 out]
                      }
                    }
                    n3163 = local read "Transaction No"() -> (w5154:string)
                    n3164 = local read "TransactionRunNo"() -> (w5156:string)
                    n3165 = call <vilib>:"Space Constant.vi"() -> ("String"=w5158:string)
                    n3166 = Concatenate Strings("{READY TO START}{RecoveryFlag=T}" ("string"), w5158, "[TransactionNo] = " ("string"), w5154, w5158, "[TransactionRunNo] = " ("string"), w5156) -> (w5152:string)
                    n3167 = call "Queue - EnQueue to MessageQ.vi"("<NoD> Don't Display to UI"=TRUE, "Message"=w5152) -> ()  [unwired: 9 in, 1 out]
                  }
                }
                n3168 = local write "RecoveryFlag"(w5095) -> ()
              }
            }
            n3169 = case shown="True" w4983 {
              frame False {
              }
              frame True {
                # "Host to maintain Folders"
                # "Folder Maintanence for Host."
                n3170 = local read "Logs_Host"() -> (w5198:path)
                n3171 = Format Date/Time String "Date_Time"(time format string (%c)="%Y%m") -> (date/time string=w5196:string)  [unwired: 2 in]
                n3172 = call "Folder - Subtract Number of Months.vi"("- # of Months"=3, "YYYYmm"=w5196, "Folder"=w5198) -> ("< Range (Folder\\YYYY\\mm)"=w5194:path[])  [unwired: 6 in, 2 out]
                n3173 = for {
                  tunnel: w5194 -> [w5200] mode=indexing
                  n3174 = Delete(path (use dialog)=w5200, entire hierarchy (F)=TRUE) -> ()  [unwired: 3 in, 3 out]
                }
              }
            }
          }
        }
        n3175 = case shown="False" w4386 {
          frame False {
            # "1st Time"
            n3176 = call "Queue - EnQueue to MessageQ.vi"("<NoD> Don't Display to UI"=TRUE, "Message"="{Ready to Start}" ("element")) -> ()  [unwired: 9 in, 1 out]
          }
          frame True {
            # "Repeating READY TO START"
          }
        }
        n3177 = Wait Until Next ms Multiple(millisecond multiple=u32 100) -> ()  [unwired: 1 out]
        n3178 = local read "Recipe Start Flag"() -> (w4384:bool)
        n3179 = case shown="False" w4384 {
          tunnel: w4383 -> [w4400 _]
          tunnel: [w4399 Enum_-_SRTRS_State."START Recipe" ("Enum")] -> w4382
          frame False {
            n3180 = case shown="False" w4400 {
              tunnel: [Enum_-_SRTRS_State."READY TO START" ("Enum") Enum_-_SRTRS_State."START Recovery" ("Enum")] -> w4399
              frame False {
              }
              frame True {
                # "DAQ Started"
              }
            }
          }
          frame True {
          }
        }
      }
      frame "START Recipe" {
        w5225 = T35 [enum."Page Disabled & Grayed", enum."Page Enabled", enum."Page Disabled & Grayed", enum."Page Disabled & Grayed", enum."Page Enabled"] items=["Page Enabled", "Page Disabled", "Page Disabled & Grayed"]
        w5203 = FALSE ("Recipe Start Flag")
        w5238 = Enum_-_SRTRS_State."BEGIN Process"  # Skip Start Recovery  (Of course!!)
        # "User has Clicked on START which\nSets the Recipe Start Flag, we will\nReset it here."
        # "If its a recovery system, there should already be one."
        # "No need existing TransactionRunNo becuase we will be\ngetting one from GetNewTransactionRunNo"
        # "Create Logging Files\nInitialise EXECUTE TAB \nINSERT [SRTRS].[Execute].[Header], ...[TransactionResult], ...[ProcedureItem]\nINSERT [CMS].[Execute].[ActivedProcess]"
        n3181 = Get Date/Time In Seconds() -> (seconds since 1Jan1904=w5212:timestamp)
        n3182 = local read "Transaction No"() -> (w5215:string)
        n3183 = property on="Tab Body" class="TabCtl (strict)"() -> ("Pages"=w5226:refnum<vi>[])  [unwired: 2 in, 2 out]
        n3184 = Bundle By Name(cluster=T19 {"TransactionNo"="", "TransactionRunNo"=""} ("Transaction"), "TransactionNo"=w5215, "TransactionRunNo"="") -> (w5214:T19)
        n3185 = Format Date/Time String(time format string (%c)="%Y%m%d_%H%M%S", seconds (now)=w5212) -> (date/time string=w5231:string)  [unwired: 1 in]
        n3186 = local read "Data_Host"() -> (w5219:path)
        n3187 = call "Folder - Create Year-Month.vi"("Folder Name"=w5219) -> ("error out"=w5218:errorcluster, "Folder with Year\\Month"=w5217:path)  [unwired: 9 in]
        n3188 = for {
          tunnel: w5226 -> [w5376] mode=indexing
          tunnel: w5225 -> [w5375] mode=indexing
          n3189 = property class="Page"(reference=w5376, "PageEnb"=w5375) -> ()  [unwired: 1 in, 2 out]
        }
        n3190 = property on="Close" class="Bool (strict)"("DisabledEnum"=T30."Disabled and Grayed Out" ("Disabled")) -> ()  [unwired: 2 in, 2 out]
        n3191 = Concatenate Strings(w5215, "_" ("string"), w5231, ".dat" ("string")) -> (w5227:string)
        n3192 = Build Path(base path=w5217, name or relative path=w5227) -> (appended path=w5209:path)
        n3193 = disable-structure shown="Disabled" {
          frame Disabled {
            n3194 = local read "Tab Body"() -> ()  [unwired: 1 in]
          }
          frame Enabled {
          }
        }
        n3195 = local write "Recipe Start Flag"(w5203) -> ()
        n3196 = Path To String(path=w5209) -> (string=w5207:string)
        n3197 = local write "Manual Stop"(w5203) -> ()
        n3198 = flat-sequence "EXECUTE TAB" {
          frame #0 {
            w5345 = T36 [{"Color Box"=9868950, "Color Box 2"=9868950}, {"Color Box"=6618880, "Color Box 2"=6618880}, {"Color Box"=4934475, "Color Box 2"=4934475}, {"Color Box"=6618880, "Color Box 2"=6618880}]  # Init
            w5346 = T36 [{"Color Box"=9868950, "Color Box 2"=9868950}, {"Color Box"=6618880, "Color Box 2"=6618880}, {"Color Box"=4934475, "Color Box 2"=4934475}, {"Color Box"=6618880, "Color Box 2"=6618880}]  # Init
            w5348 = cluster{"Color Box":u32, "Color Box 2":u32}[] [{"Color Box"=16383786, "Color Box 2"=16383786}, {"Color Box"=6618880, "Color Box 2"=6618880}, {"Color Box"=4934475, "Color Box 2"=4934475}, {"Color Box"=6618880, "Color Box 2"=6618880}]  # Start Recipe
            w5360 = timestamp(3471350400 s since 1904-01-01) ("Parameter (Start Dwell Time)")
            # "0 - do not autoscale,\n1 - autoscale once now, or \n2 - autoscale."
            # "\"Start Recipe\""
            n3199 = local write "Parameter (Start Dwell Time)"(w5360) -> ()
            n3200 = local write "% Hold. Time Completed (Num)"(0.0 ("% Hold. Time Completed (Num)")) -> ()
            n3201 = local write "Parameter (End Dwell Time)"(w5360) -> ()
            n3202 = property on="% Hold. Time Completed" class="Slide (strict)"("Scale.Maximum"=100.0 ("Scale.Range:Maximum"), "Scale.Minimum"=0.0 ("Scale.Range:Minimum"), "Fill Color"=u32 16777216 ("Color Box 2"), "Value"=0.0 ("% Hold Time Completed")) -> ()  [unwired: 2 in, 2 out]
            n3203 = property on="Variant Allowed (Hold Temp)" class="Bool (strict)"("Colors [4]"=w5346, "Value"=FALSE) -> ()  [unwired: 2 in, 2 out]
            n3204 = property on="Variant Allowed (Hold Time)" class="Bool (strict)"("Colors [4]"=w5346, "Value"=FALSE) -> ()  [unwired: 2 in, 2 out]
            n3205 = property on="Hold. Time (hour:minute)" class="Str"() -> ("Value"=w5356:string)  [unwired: 2 in, 2 out]
            n3206 = call "String - Format to (HH_colon_MM).vi"("xx:xx"=w5356) -> ("seconds"=w5354:dbl)  [unwired: 9 in, 1 out]
            n3207 = flat-sequence {
              frame #0 {
                w5364 = 12  # 12 Probes Max
